vi "KE622x -- 2182 -A Write tmp.vi"(0 "Resource In":refnum<visa-resource-name>, 1 "Check For SCPI Errors? (T)":bool=TRUE, 7 "2182-A Write String":string, 11 "error in (no error)":errorcluster) -> (4 "Resource Out (dupl)":refnum<visa-resource-name>, 15 "error out":errorcluster)   [LabVIEW 2014, in "Keithley 622x tmp.lvlib"]
uses:
  Keithley 622x tmp.lvlib
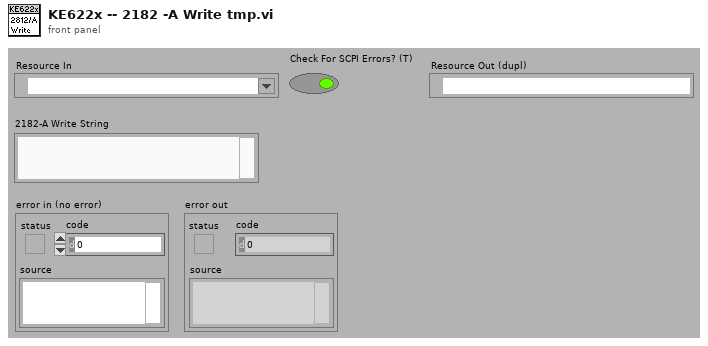
[diagram p1: front panel]
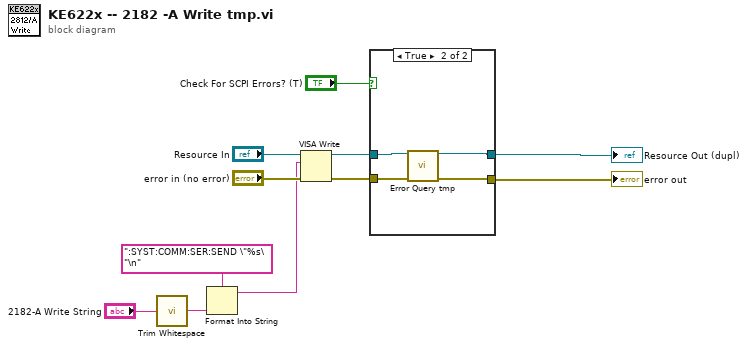
[diagram p0: block diagram]
diagram:
  n1 = call <vilib>:"Trim Whitespace.vi"("string"="2182-A Write String") -> ("trimmed string"=w2:string)  [unwired: 1 in]
  n2 = Format Into String(format string=":SYST:COMM:SER:SEND \"%s\"\n", w2) -> (resulting string=w1:string)  [unwired: 2 in, 1 out]
  n3 = VISA Write(VISA resource name="Resource In", write buffer=w1, error in (no error)="error in (no error)") -> (VISA resource name out=w8:refnum<visa-resource-name>, error out=w7:errorcluster)  [unwired: 1 out]
  n4 = case shown="True" "Check For SCPI Errors? (T)" {
    tunnel: w8 -> [w13 w17]
    tunnel: w7 -> [w12 w16]
    tunnel: [w12 w14] -> w5
    tunnel: [w13 w15] -> w6
    frame False {
    }
    frame True {
      n5 = call "Error Query tmp.vi"("VISA Resource In"=w17, "error in (no error)"=w16) -> ("VISA Resource Out (dupl)"=w15:refnum<visa-resource-name>, "error out"=w14:errorcluster)  [unwired: 10 in, 2 out]
    }
  }
  "Resource Out (dupl)" <- w6
  "error out" <- w5
